vi "RMS (DBL).vi"(0 "X":dbl[](array[numeric]) format="%0.2f") -> (1 "rms value":dbl format="%0.2f", 2 "error":i32)   [LabVIEW 2022 SP3, in "NI_AALPro.lvlib"]
doc: "Computes the root mean square (rms) of the input sequence <B>X</B>."
uses:
  NI_AALPro.lvlib
  <resource>/lvanlys.dll
panel:
  # "RMS"
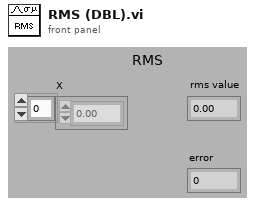
[diagram p1: front panel]
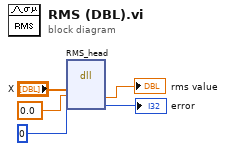
[diagram p0: block diagram]
diagram:
  n1 = dll-call lib="C:/Program Files (x86)/National Instruments/LabVIEW 2022/resource/lvanlys.*" fn="RMS_head"("X"="X", "output param"=0.0, "output param"=0) -> ("output param"=→"rms value":dbl, "output param"=→"error":i32)  [unwired: 5 in, 2 out]
